vi "Find Static Test Methods.vi"(8 "error in (no error)":errorcluster, 10 "Test Methods In":map{string, path}(c390), 11 "LVClassLibrary in":refnum<vi>) -> (0 "error out":errorcluster, 2 "Test Methods Out":map{string, path}(c390), 3 "LVClassLibrary out":refnum<vi>)   [LabVIEW 2020, in "Test Finder.lvclass"]
uses:
  Test Finder.lvclass
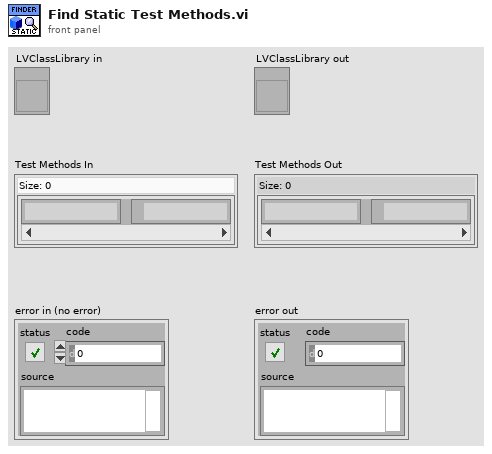
[diagram p1: front panel]
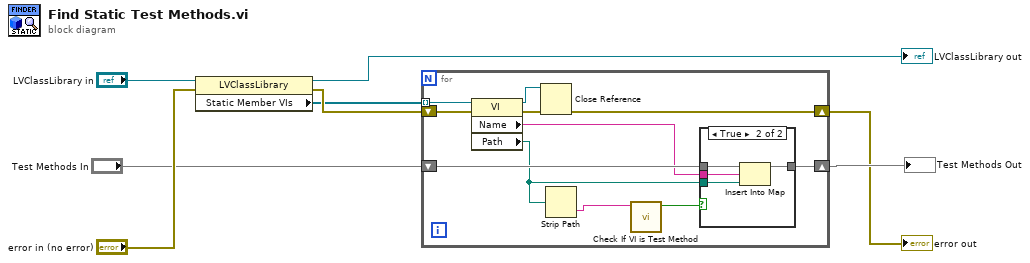
[diagram p0: block diagram]
diagram:
  n1 = property class="LVClassLibrary"(reference="LVClassLibrary in", error in="error in (no error)") -> (reference out=→"LVClassLibrary out":refnum<vi>, error out=w5:errorcluster, "Static Member VIs"=w4:refnum<vi>[])
  n2 = for {
    tunnel: w4 -> [w19] mode=indexing
    shift-right: [w15] -> w1
    shift-left: w5 -> [w18]
    shift-right: [w13] -> w2
    shift-left: "Test Methods In" -> [w14]
    n3 = property class="VI"(reference=w19, error in=w18) -> (reference out=w16:refnum<vi>, error out=w17:errorcluster, "Name"=w12:string, "Path"=w10:path)
    n4 = Close Reference(reference=w16, error in (no error)=w17) -> (error out=w15:errorcluster)
    n5 = Strip Path(path=w10) -> (name=w9:string)  [unwired: 1 out]
    n6 = call "Check If VI is Test Method.vi"("VI Name"=w9) -> ("Is Test Method?"=w11:bool)  [unwired: 9 in, 1 out]
    n7 = case shown="True" w11 {
      tunnel: w14 -> [w20 w24]
      tunnel: w10 -> [_ w23]
      tunnel: [w20 w22] -> w13
      tunnel: w12 -> [_ w21]
      frame False {
      }
      frame True {
        n8 = Insert Into Map(map in=w24, key=w21, value=w23) -> (map out=w22:map{string, path})  [unwired: 2 out]
      }
    }
  }
  "error out" <- w1
  "Test Methods Out" <- w2
